vi "CloseLidar.vi"(8 "error in (no error)":errorcluster, 11 "VISA Refnum in":refnum<visa-resource-name>) -> (0 "error out":errorcluster)   [LabVIEW 2016]
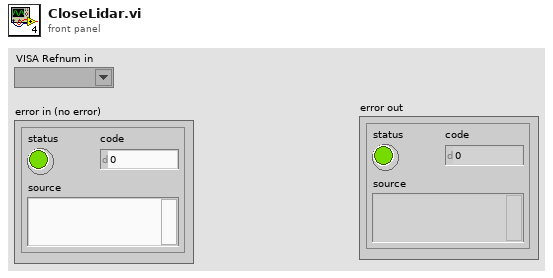
[diagram p1: front panel]
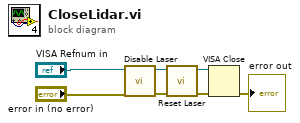
[diagram p0: block diagram]
diagram:
  n1 = call "Disable Laser.vi"("error in (no error)"="error in (no error)", "VISA Refnum in"="VISA Refnum in") -> ("error out"=w2:errorcluster, "VISA Refnum out"=w4:refnum<visa-resource-name>)  [unwired: 8 in]
  n2 = call "Reset Laser.vi"("error in (no error)"=w2, "VISA Refnum in"=w4) -> ("error out"=w3:errorcluster, "VISA Refnum out"=w5:refnum<visa-resource-name>)  [unwired: 8 in]
  n3 = VISA Close(VISA resource name=w5, error in (no error)=w3) -> (error out=→"error out":errorcluster)
